vi "Controller Test Bench (8).vi"() -> ()   [LabVIEW 2022 SP3]
uses:
  <vilib>/sound2/lvsound2.llb/Sound Data Format.ctl
  <vilib>/Utility/error.llb/DialogType.ctl
  <vilib>/sound2/lvsound2.llb/Sampling Mode.ctl
  <vilib>/Analysis/4window.llb/windowTd.ctl
  <vilib>/DAQmx/read.llb/DAQmx Read (Analog 1D Wfm NChan NSamp).vi
  <vilib>/DAQmx/write.llb/DAQmx Write (Analog 1D DBL 1Chan NSamp).vi
  <vilib>/DAQmx/create/channels.llb/DAQmx Create Channel (AO-Voltage-Basic).vi
  <vilib>/DAQmx/create/channels.llb/DAQmx Create Channel (AI-Acceleration-Accelerometer).vi
  <vilib>/DAQmx/configure/timing.llb/DAQmx Timing (Sample Clock).vi
  <vilib>/DAQmx/miscellaneous.llb/DAQmx Fill In Error Info.vi
  <vilib>/DAQmx/configure/task.llb/DAQmx Configure Logging (TDMS).vi
  <vilib>/measure/maspectr.llb/FFT Spectrum (Mag-Phase) for N Chan.vi
  <vilib>/sound2/lvsound2.llb/Sound Output Set Volume (Single).vi
  <vilib>/sound2/lvsound2.llb/Sound Output Write (DBL Single).vi
  <vilib>/measure/NI_MAPro.lvlib
  <resource>/objmgr/daqmx.rc
  <vilib>/Analysis/NI_AALPro.lvlib
  <vilib>/measure/NI_MABase.lvlib
panel:
  out "Waveform Chart":waveform(dbl)[](graph)
  out "Accel.1":waveform(dbl)[](graph)
  out "Accel.2":waveform(dbl)[](graph)
  in  "Setpoint":dbl
  in  "Gain":dbl min=0.0 step=0.01
  out "Numeric":i32
  in  "Output Noise":bool
  in  "reset signal":bool
  out "number of samples written per channel":u32
  in  "Active Control":bool
  in  "Log Data":bool
  out "Phase 2":cluster{"f0":dbl, "df":dbl, "phase":dbl[]}[](graph)
  out "Mag 2":cluster{"f0":dbl, "df":dbl, "magnitude":dbl[]}[](graph)
  in  "Show FFT":bool
  in  "Save FFT":bool
  in  "Start Acquisition":bool
  in  "Stop":bool
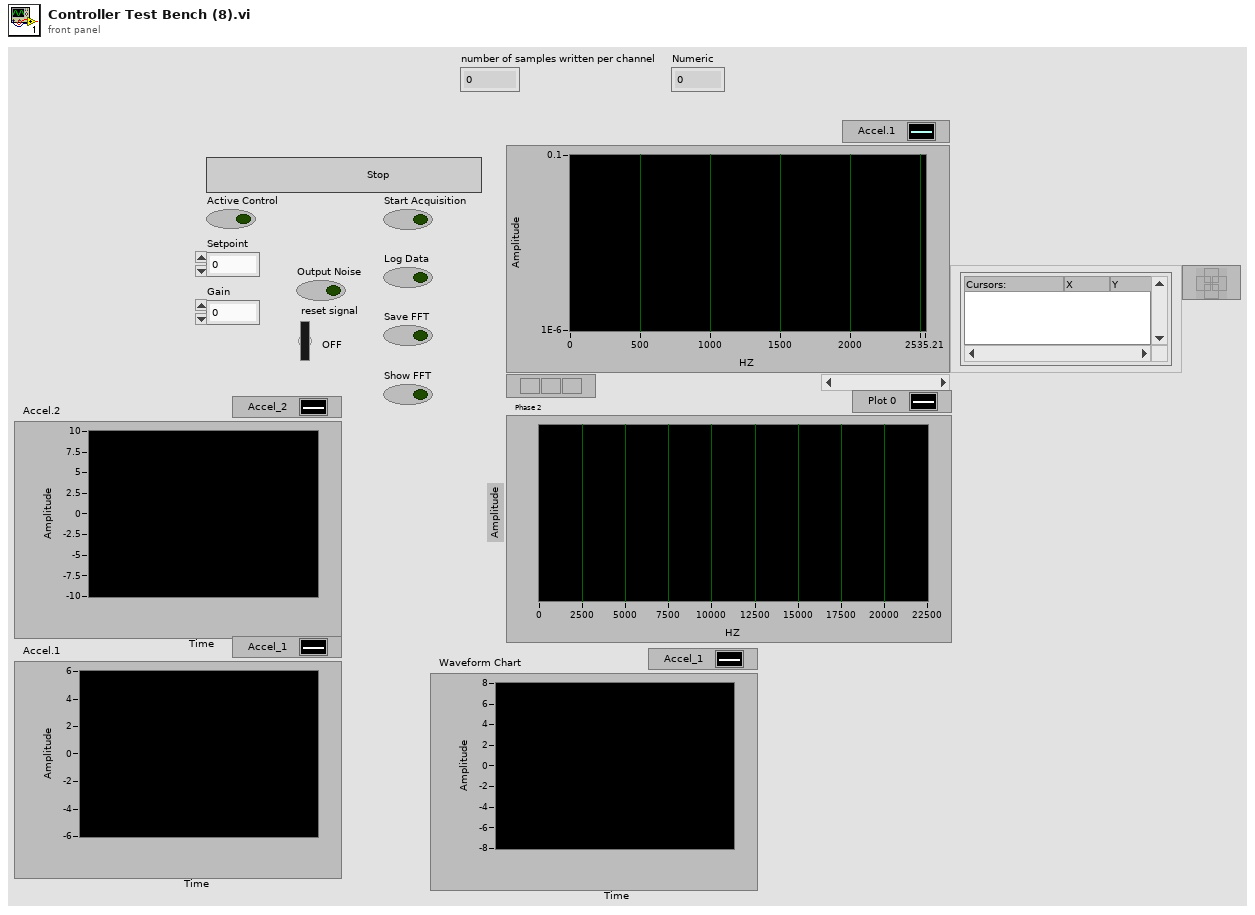
[diagram p1: front panel]
types:
  T1 = typedef "Sampling Mode.ctl" = i32
  T2 = typedef "DialogType.ctl" = u16
  T3 = typedef "Sound Data Format.ctl" = cluster{"sample rate (S/s)":dbl, "number of channels":i32, "bits per sample":i32}
  T4 = typedef "Sound Output Task ID.ctl" = u32
  T5 = typedef "NI_AALPro.lvlib/windowTd.ctl" = u32
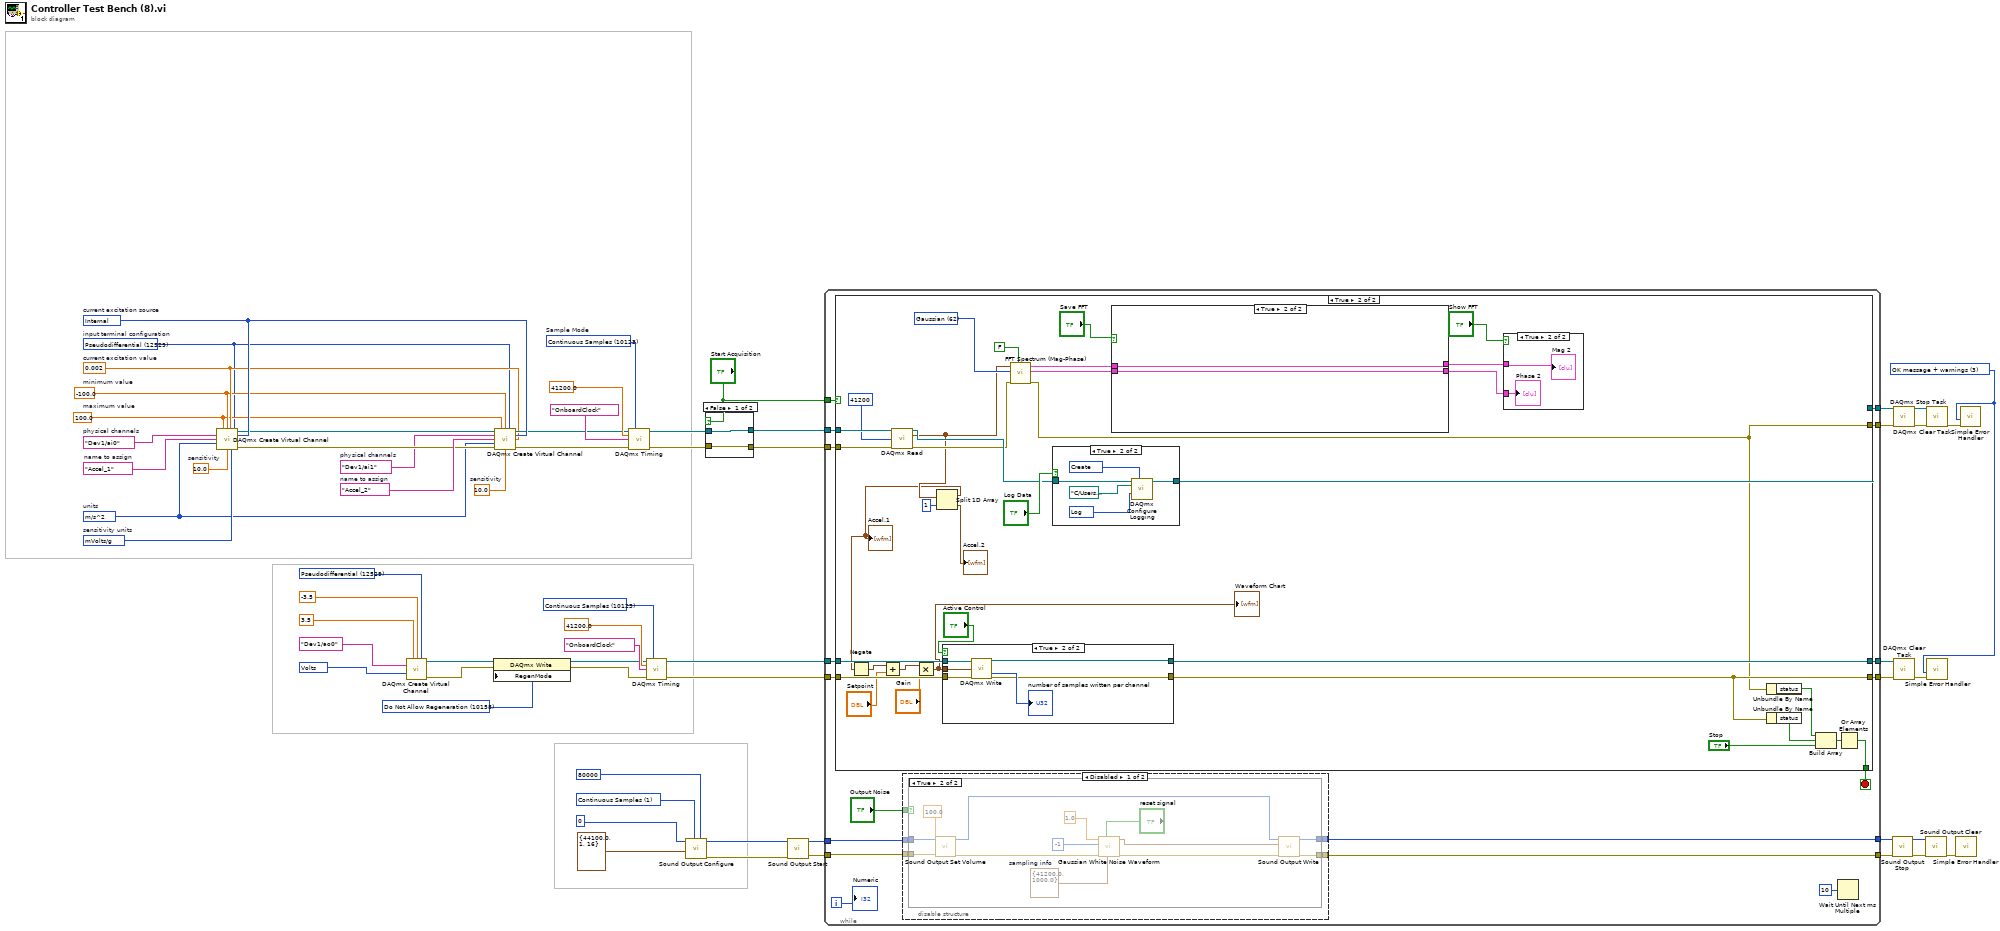
[diagram p0: block diagram]
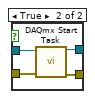
[diagram p2: hidden frame]
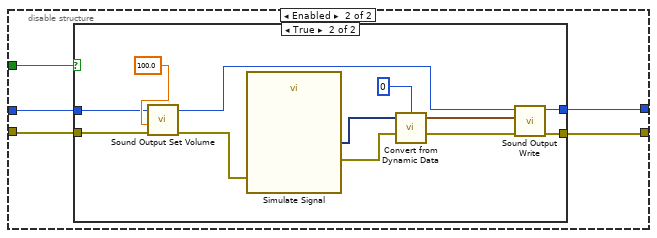
[diagram p4: hidden frame]
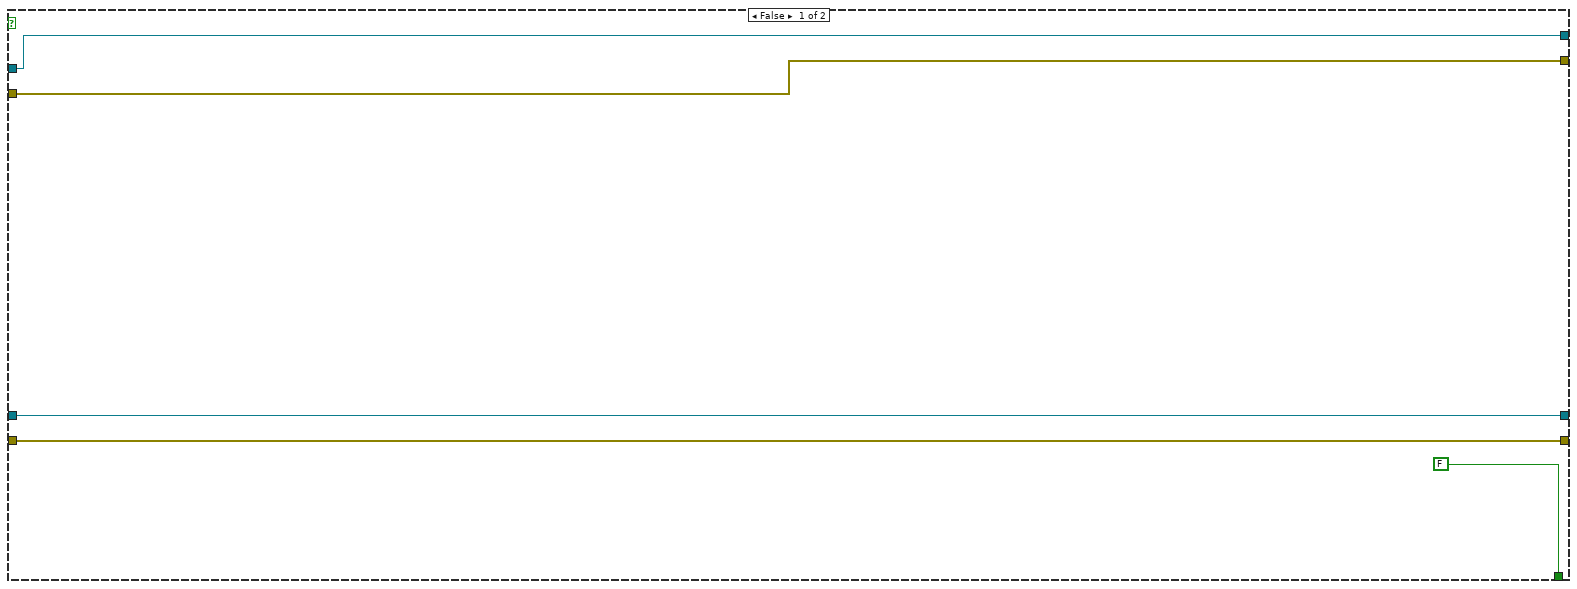
[diagram p6: hidden frame]
diagram:
  w25 = 10123 items=["Finite Samples"=10178, "Continuous Samples"=10123, "Hardware Timed Single Point"=12522] ("sample mode")
  w29 = 12509 items=["mVolts/g"=12509, "Volts/g"=12510]  # sensitivity units
  w30 = 10.0  # sensitivity
  w19 = 0.002  # current excitation value
  w22 = 10200 items=["Internal"=10200, "External"=10167, "None"=10230]  # current excitation source
  w12 = tag "Dev1/ai0"  # physical channels
  w28 = 10123 items=["Finite Samples"=10178, "Continuous Samples"=10123, "Hardware Timed Single Point"=12522]  # Sample Mode
  w15 = 12529 items=["default"=-1, "RSE"=10083, "NRSE"=10078, "Differential"=10106, "Pseudodifferential"=12529]  # input terminal configuration
  w18 = -100.0  # minimum value
  w17 = 100.0  # maximum value
  w31 = "Accel_1"  # name to assign
  w16 = 12470 items=["g"=10186, "m/s^2"=12470, "in/s^2"=12471, "From Custom Scale"=10065]  # units
  w32 = 10.0  # sensitivity
  w13 = tag "Dev1/ai1"  # physical channels
  w24 = "Accel_2"  # name to assign
  w33 = T1 1 items=["Finite Samples", "Continuous Samples"] ("sample mode")
  w44 = 10158 items=["Allow Regeneration"=10097, "Do Not Allow Regeneration"=10158] ("RegenMode")
  w34 = T2 3 items=["no dialog", "OK message", "continue or stop message", "OK message + warnings", "continue/stop + warnings"] ("type of dialog (OK msg:1)")
  w57 = 12529 items=["Default"=-1, "RSE"=10083, "Differential"=10106, "Pseudodifferential"=12529] ("output terminal configuration")
  w55 = 10348 items=["Volts"=10348, "From Custom Scale"=10065] ("units")
  n1 = call-poly <vilib>:"DAQmx Create Virtual Channel.vi"("maximum value"=w17, "minimum value"=w18, "input terminal configuration"=w15, "physical channels"=w12, "current excitation source"=w22, "name to assign"=w31, "current excitation value"=w19, "units"=w16, "sensitivity"=w30, "sensitivity units"=w29) -> ("task out"=w14:refnum<k21>, "error out"=w23:errorcluster)  [unwired: 4 in]
  n2 = call-poly <vilib>:"DAQmx Create Virtual Channel.vi"("maximum value"=3.5, "minimum value"=-3.5, "output terminal configuration"=w57, "physical channels"=tag "Dev1/ao0", "units"=w55) -> ("task out"=w41:refnum<k21>, "error out"=w45:errorcluster)  [unwired: 9 in]
  n3 = property class="DAQmx Write"(reference=w41, error in=w45, "RegenMode"=w44) -> (reference out=w39:refnum<k21>, error out=w40:errorcluster)
  n4 = call-poly <vilib>:"DAQmx Create Virtual Channel.vi"("task in"=w14, "maximum value"=w17, "minimum value"=w18, "input terminal configuration"=w15, "physical channels"=w13, "current excitation source"=w22, "name to assign"=w24, "current excitation value"=w19, "units"=w16, "error in"=w23, "sensitivity"=w32) -> ("task out"=w21:refnum<k21>, "error out"=w20:errorcluster)  [unwired: 3 in]
  n5 = call-poly <vilib>:"DAQmx Timing.vi"("task/channels in"=w21, "sample mode"=w28, "rate"=41200.0 ("Sample Rate"), "source"=tag "OnboardClock" ("Sample Clock Source"), "error in"=w20) -> ("task out"=w10:refnum<k21>, "error out"=w11:errorcluster)  [unwired: 9 in]
  n6 = call-poly <vilib>:"DAQmx Timing.vi"("task/channels in"=w39, "sample mode"=w25, "rate"=41200.0 ("Sample Rate"), "source"=tag "OnboardClock" ("Sample Clock Source"), "error in"=w40) -> ("task out"=w43:refnum<k21>, "error out"=w42:errorcluster)  [unwired: 9 in]
  n7 = call <vilib>:"Sound Output Configure.vi"("number of samples/ch"=80000 ("Number of Samples/ch"), "sample mode"=w33, "sound format"=T3 {"sample rate (S/s)"=44100.0, "number of channels"=1, "bits per sample"=16} ("Sound Format"), "device ID"=u32 0 ("Device ID")) -> ("error out"=w2:errorcluster, "task ID"=w1:T4)  [unwired: 6 in]
  n8 = case shown="False" "Start Acquisition" {
    tunnel: w11 -> [w63 w68]
    tunnel: w10 -> [w64 w67]
    tunnel: [w64 w66] -> w54
    tunnel: [w63 w65] -> w53
    frame False {
    }
    frame True {
      n9 = call <vilib>:"DAQmx Start Task.vi"("task/channels in"=w67, "error in"=w68) -> ("task out"=w66:refnum<k21>, "error out"=w65:errorcluster)  [unwired: 12 in]
    }
  }
  n10 = call <vilib>:"Sound Output Start.vi"("error in (no error)"=w2, "task ID"=w1) -> ("error out"=w3:errorcluster, "task ID out"=w4:T4)  [unwired: 8 in]
  n11 = while {
    tunnel: w3 -> [w73]
    tunnel: w4 -> [w74]
    tunnel: w54 -> [w84]
    tunnel: w53 -> [w83]
    tunnel: [w81] -> w49
    tunnel: [w82] -> w48
    tunnel: w43 -> [w80]
    tunnel: w42 -> [w79]
    tunnel: [w77] -> w38
    tunnel: [w78] -> w37
    tunnel: "Start Acquisition" -> [w76]
    tunnel: [w71] -> w6
    tunnel: [w70] -> w5
    i -> [w72]
    stop <- w85 stop-if-true
    n12 = case shown="True" w76 {
      tunnel: [FALSE w163] -> w85
      tunnel: w84 -> [w128 w162]
      tunnel: w83 -> [w127 w161]
      tunnel: [w128 w158] -> w82
      tunnel: [w127 w142] -> w81
      tunnel: w80 -> [w126 w148]
      tunnel: w79 -> [w125 w147]
      tunnel: [w126 w146] -> w78
      tunnel: [w125 w145] -> w77
      frame False {
      }
      frame True {
        w141 = T5 62 items=["Rectangle"=0, "Hanning"=1, "Hamming"=2, "Blackman-Harris"=3, "Exact Blackman"=4, "Blackman"=5, "Flat Top"=6, "4 Term B-Harris "=7, "7 Term B-Harris"=8, "Low Sidelobe"=9, "Blackman Nuttall"=11, "Triangle"=30, "Bartlett-Hanning"=31, "Bohman"=32, "Parzen"=33, "Welch"=34, "Kaiser"=60, "Dolph-Chebyshev"=61, "Gaussian"=62] ("window")
        n13 = call-poly <vilib>:"DAQmx Read.vi"("task/channels in"=w162, "number of samples per channel"=41200, "error in"=w161) -> ("task out"=w159:refnum<k21>, "data"=w134:waveform(dbl)[], "error out"=w143:errorcluster)  [unwired: 10 in]
        n14 = Split 1D Array(array=w134, index=1) -> (first subarray=w129:waveform(dbl)[], second subarray=→"Accel.2":waveform(dbl)[])
        "Accel.1" <- w129
        n15 = Negate(x=w129) -> (-x=w136:waveform(dbl)[])
        n16 = Add(x=w136, y="Setpoint") -> (x+y=w137:waveform(dbl)[])
        n17 = Multiply(x=w137, y="Gain") -> (x*y=w130:waveform(dbl)[])
        "Waveform Chart" <- w130
        n18 = case shown="True" "Active Control" {
          tunnel: w147 -> [w165 w169]
          tunnel: [w164 w166] -> w146
          tunnel: [w165 w167] -> w145
          tunnel: w148 -> [w164 w171]
          tunnel: w130 -> [_ w170]
          frame False {
          }
          frame True {
            n19 = call-poly <vilib>:"DAQmx Write.vi"("task/channels in"=w171, "data"=w170, "error in"=w169) -> ("task out"=w166:refnum<k21>, "number of samples written per channel"=→"number of samples written per channel":u32, "error out"=w167:errorcluster)  [unwired: 10 in]
          }
        }
        n20 = call-poly <vilib>:"FFT Spectrum (Mag-Phase).vi"("restart averaging (F)"=FALSE, "error in (no error)"=w143, "window"=w141, "time signals"=w134) -> ("error out"=w142:errorcluster, "phases"=w152:cluster{"f0":dbl, "df":dbl, "phase":dbl[]}[], "magnitudes"=w153:cluster{"f0":dbl, "df":dbl, "magnitude":dbl[]}[])  [unwired: 3 in, 2 out]
        n21 = case shown="True" "Log Data" {
          tunnel: w159 -> [w178 w180]
          tunnel: [w178 w179] -> w158
          frame False {
          }
          frame True {
            w181 = 15848 items=["Open"=10437, "Open or Create"=15846, "Create or Replace"=15847, "Create"=15848] ("operation")
            w182 = 15844 items=["Off"=10231, "Log"=15844, "Log and Read"=15842] ("logging mode")
            n22 = call-poly <vilib>:"DAQmx Configure Logging.vi"("task/channels in"=w180, "operation"=w181, "file path"=path "C:/Users/LAV-UFSC/Documents/LAV - TCC", "logging mode"=w182) -> ("task out"=w179:refnum<k21>)  [unwired: 10 in, 1 out]
          }
        }
        n23 = case shown="True" "Save FFT" {
          tunnel: w153 -> [w172 w175]
          tunnel: w152 -> [w173 w174]
          tunnel: [w173 w174] -> w151
          tunnel: [w172 w175] -> w150
          frame False {
          }
          frame True {
          }
        }
        n24 = case shown="True" "Show FFT" {
          tunnel: w150 -> [_ w177]
          tunnel: w151 -> [_ w176]
          frame False {
          }
          frame True {
            "Mag 2" <- w177
            "Phase 2" <- w176
          }
        }
        n25 = Unbundle By Name(w142) -> ("status"=w139:bool)
        n26 = Unbundle By Name(w145) -> ("status"=w149:bool)
        n27 = Build Array(w139, w149, "Stop") -> (w156:bool[])
        n28 = Or Array Elements(Boolean array=w156) -> (logical OR=w163:bool)
      }
    }
    n29 = disable-structure shown="Disabled" {
      disable-tunnel: "Output Noise" -> [w90 w110]
      disable-tunnel: w74 -> [w89 w108]
      disable-tunnel: w73 -> [w88 w109]
      disable-tunnel: [w87 w107] -> w71
      disable-tunnel: [w86 w106] -> w70
      frame Disabled {
        n30 = case shown="True" w90 {
          tunnel: w88 -> [w91 w102]
          tunnel: w89 -> [w92 w103]
          tunnel: [w92 w105] -> w86
          tunnel: [w91 w104] -> w87
          frame False {
          }
          frame True {
            w93 = cluster{"Fs":dbl, "#s":dbl} {"Fs"=41200.0, "#s"=1000.0}  # sampling info
            n31 = call-poly <vilib>:"Sound Output Set Volume.vi"("error in (no error)"=w102, "volume"=100.0, "task ID"=w103) -> ("error out"=w99:errorcluster, "task ID out"=w101:T4)  [unwired: 7 in]
            n32 = call <vilib>:"Gaussian White Noise Waveform.vi"("sampling info"=w93, "reset signal"="reset signal", "error in (no error)"=w99, "seed"=-1, "standard deviation"=1.0) -> ("error out"=w98:errorcluster, "signal out"=w97:waveform(dbl))  [unwired: 5 in]
            n33 = call-poly <vilib>:"Sound Output Write.vi"("error in (no error)"=w98, "data"=w97, "task ID"=w101) -> ("error out"=w104:errorcluster, "task ID out"=w105:T4)  [unwired: 7 in]
          }
        }
      }
      frame Enabled {
        n34 = case shown="True" w110 {
          tunnel: w109 -> [w112 w116]
          tunnel: w108 -> [w111 w115]
          tunnel: [w112 w114] -> w107
          tunnel: [w111 w113] -> w106
          frame False {
          }
          frame True {
            n35 = call-poly <vilib>:"Sound Output Set Volume.vi"("error in (no error)"=w116, "volume"=100.0, "task ID"=w115) -> ("error out"=w121:errorcluster, "task ID out"=w120:T4)  [unwired: 7 in]
            n36 = call "Simulate Signal"("error in (no error)"=w121) -> ("DC with Gaussian Noise"=w123:dynamicdata, "error out"=w117:errorcluster)  [unwired: 13 in]
            n37 = call "Convert from Dynamic Data"("Dynamic Data Type"=w123, "Channel"=0) -> ("Waveform"=w122:waveform(dbl))  [unwired: 2 in]
            n38 = call-poly <vilib>:"Sound Output Write.vi"("error in (no error)"=w117, "data"=w122, "task ID"=w120) -> ("error out"=w114:errorcluster, "task ID out"=w113:T4)  [unwired: 7 in]
          }
        }
      }
    }
    n39 = Wait Until Next ms Multiple(millisecond multiple=u32 10) -> ()  [unwired: 1 out]
    "Numeric" <- w72
  }
  n40 = call <vilib>:"Sound Output Stop.vi"("error in (no error)"=w6, "task ID"=w5) -> ("error out"=w9:errorcluster, "task ID out"=w8:T4)  [unwired: 8 in]
  n41 = call <vilib>:"DAQmx Stop Task.vi"("task/channels in"=w48, "error in"=w49) -> ("task out"=w51:refnum<k21>, "error out"=w50:errorcluster)  [unwired: 12 in]
  n42 = call <vilib>:"DAQmx Clear Task.vi"("task in"=w37, "error in"=w38) -> ("error out"=w36:errorcluster)  [unwired: 13 in]
  n43 = call <vilib>:"Sound Output Clear.vi"("error in (no error)"=w9, "task ID"=w8) -> ("error out"=w7:errorcluster)  [unwired: 9 in]
  n44 = call <vilib>:"DAQmx Clear Task.vi"("task in"=w51, "error in"=w50) -> ("error out"=w52:errorcluster)  [unwired: 13 in]
  n45 = call <vilib>:"Simple Error Handler.vi"("type of dialog (OK msg:1)"=w34, "error in (no error)"=w36) -> ()  [unwired: 3 in, 5 out]
  n46 = call <vilib>:"Simple Error Handler.vi"("error in (no error)"=w7) -> ()  [unwired: 4 in, 5 out]
  n47 = call <vilib>:"Simple Error Handler.vi"("type of dialog (OK msg:1)"=w34, "error in (no error)"=w52) -> ()  [unwired: 3 in, 5 out]
